vi "ReadABF.vi"(4 "Error IN":errorcluster caption="에러 입력", 6 "FilePath":path=path "C:/Users/KimYG/Experimental Data/Flocculus_Ex vivo/6. Plsticity/190119/190119_#07/190119__0026.abf", 7 "ABFFIO.lvclass IN":refnum<class "ABFFIO.lvclass">) -> (0 "Error OUT":errorcluster caption="에러 출력", 3 "ABFFIO.lvclass OUT":refnum<class "ABFFIO.lvclass">)   [LabVIEW 2017, in "ABFFIO.lvclass"]
uses:
  ABFFIO.lvclass
  ABFFIO.lvclass/ABFFIO.ctl
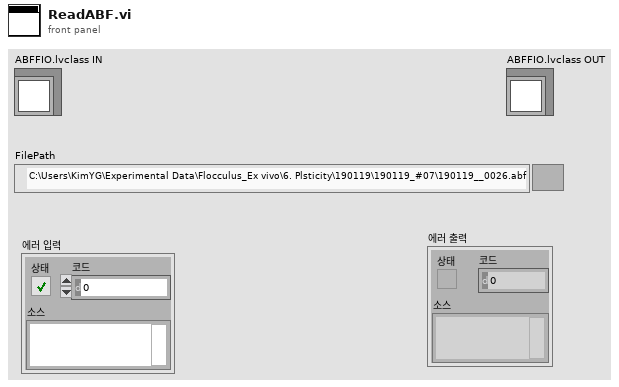
[diagram p1: front panel]
types:
  T1 = enum16{"open", "replace", "create", "open or create", "replace or create", "replace or create with confirmation"}
  T2 = enum16{"big-endian, network order", "native, host order", "little-endian"}
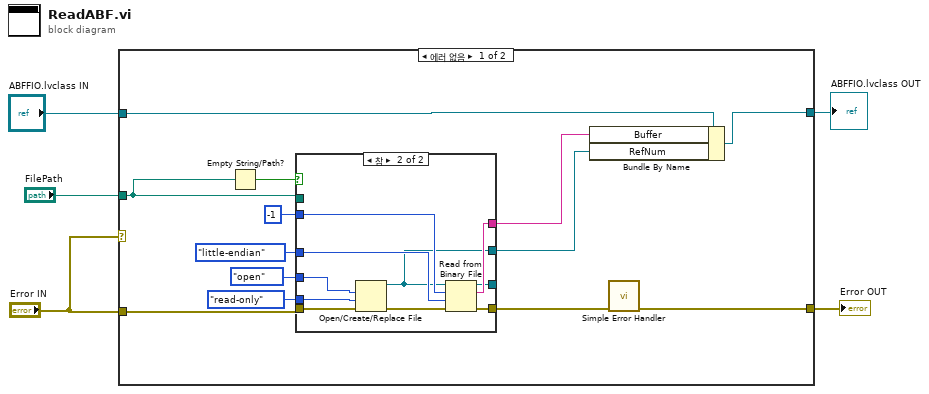
[diagram p0: block diagram]
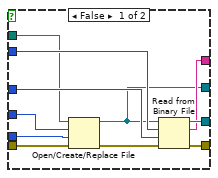
[diagram p2: hidden frame]
diagram:
  n1 = case shown="에러 없음" "Error IN" {
    tunnel: "ABFFIO.lvclass IN" -> [w14 _]
    tunnel: [w12 _] -> w4
    tunnel: "Error IN" -> [w11 _]
    tunnel: [w10 _] -> w2
    tunnel: "FilePath" -> [w6 _]
    frame No Error {
      n2 = Empty String/Path?(string/path=w6) -> (empty?=w15:bool)
      n3 = case shown="참" w15 {
        tunnel: T2."little-endian" ("바이트 순서(0:big-endian, network order)") -> [w29 w38]
        tunnel: [w28 w35] -> _
        tunnel: [w27 w39] -> w17
        tunnel: w11 -> [w24 w34]
        tunnel: -1 ("numBytes") -> [w26 w37]
        tunnel: [w25 w36] -> w13
        tunnel: w6 -> [w20 _]
        tunnel: T1."open" ("operation (0:open)") -> [w22 w32]
        tunnel: enum16{"read/write", "read-only", "write-only"}."read-only" ("access (0:read/write)") -> [w21 w31]
        tunnel: [w19 w30] -> w7
        frame False {
          n4 = Open/Create/Replace File(file path (use dialog)=w20, error in=w24, operation (0:open)=w22, access (0:read/write)=w21) -> (refnum out=w19:refnum<file>, error out=w23:errorcluster)  [unwired: 2 in, 1 out]
          n5 = Read from Binary File(8:w23, 9:w29, 10:w26, 11:w19) -> (0:w27:errorcluster, 2:w25:string, 3:w28:refnum<file>)  [unwired: 2 in, 1 out]
        }
        frame True {
          n6 = Open/Create/Replace File(error in=w34, operation (0:open)=w32, access (0:read/write)=w31) -> (refnum out=w30:refnum<file>, error out=w33:errorcluster)  [unwired: 3 in, 1 out]
          n7 = Read from Binary File(8:w33, 9:w38, 10:w37, 11:w30) -> (0:w39:errorcluster, 2:w36:string, 3:w35:refnum<file>)  [unwired: 2 in, 1 out]
        }
      }
      n8 = Bundle By Name(cluster=w14, "Buffer"=w13, "RefNum"=w7) -> (w12:refnum<class "ABFFIO.lvclass">)
      n9 = call <vilib>:"Simple Error Handler.vi"("error in (no error)"=w17) -> ("error out"=w10:errorcluster)  [unwired: 4 in, 4 out]
    }
    frame Error {
    }
  }
  "ABFFIO.lvclass OUT" <- w4
  "Error OUT" <- w2
